vi "switch trend on graph (SubVI).vi"(0 "Active Plot":u32, 1 "Chart 1":refnum<vi>, 2 "is enabled?":bool, 9 "sel eference":refnum<vi>, 11 "error in":errorcluster, 12 "Chart 2":refnum<vi>) -> (15 "error out":errorcluster)   [LabVIEW 2015]
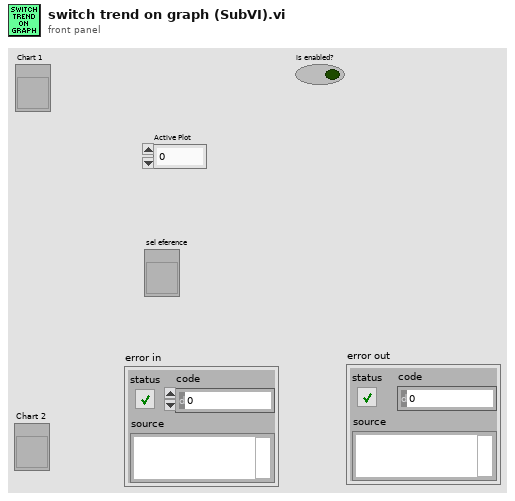
[diagram p1: front panel]
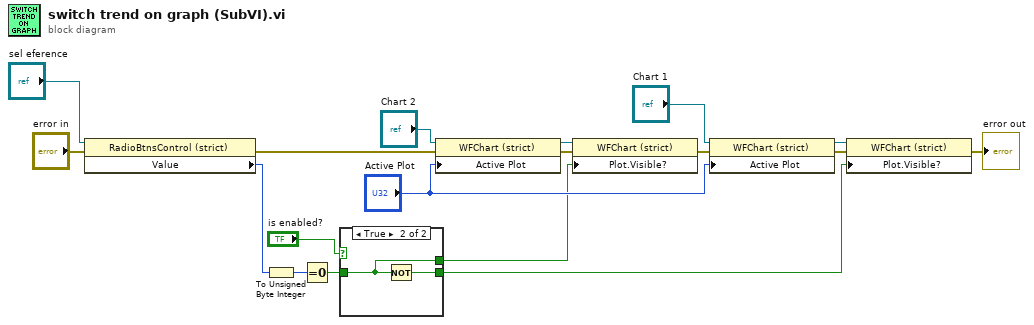
[diagram p0: block diagram]
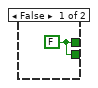
[diagram p2: hidden frame]
diagram:
  n1 = property class="RadioBtnsControl (strict)"(reference="sel eference", error in="error in") -> (error out=w7:errorcluster, "Value"=w9:enum32{"Radio Selection 1", "Radio Selection 2"})  [unwired: 1 out]
  n2 = To Unsigned Byte Integer(number=w9) -> (unsigned 8bit integer=w8:u8)
  n3 = Equal To 0?(x=w8) -> (x = 0?=w3:bool)
  n4 = case shown="True" "is enabled?" {
    tunnel: [w19 w21] -> w16
    tunnel: w3 -> [_ w20]
    tunnel: [w19 w20] -> w2
    frame False {
      w19 = FALSE
    }
    frame True {
      n5 = Not(x=w20) -> (.not. x?=w21:bool)
    }
  }
  n6 = property on="Property Node" class="WFChart (strict)"(reference="Chart 2", error in=w7, "Active Plot"="Active Plot") -> (reference out=w14:refnum<vi>, error out=w18:errorcluster)
  n7 = property on="Property Node" class="WFChart (strict)"(reference=w14, error in=w18, "Plot.Visible?"=w2) -> (error out=w12:errorcluster)  [unwired: 1 out]
  n8 = property on="Property Node" class="WFChart (strict)"(reference="Chart 1", error in=w12, "Active Plot"="Active Plot") -> (reference out=w15:refnum<vi>, error out=w17:errorcluster)
  n9 = property on="Property Node" class="WFChart (strict)"(reference=w15, error in=w17, "Plot.Visible?"=w16) -> (error out=→"error out":errorcluster)  [unwired: 1 out]
